vi "Cleanup.vi"(8 "error in (no error)":errorcluster, 11 "LabBOT in":refnum<class "LabBOT.lvclass">) -> (0 "error out":errorcluster)   [LabVIEW 2020, in "Rover.lvlib" / "LabBOT.lvclass"]
uses:
  LabBOT.lvclass
  LabBOT.lvclass/LabBOT.ctl
  Rover/Rover.lvclass
  nmea/nmea/VISA GPS/VISA GPS.lvclass
  bno055/BNO055/BNO055/BNO055.lvclass
  <vilib>/MakerHub/LINX/LMH-LINX.lvlib
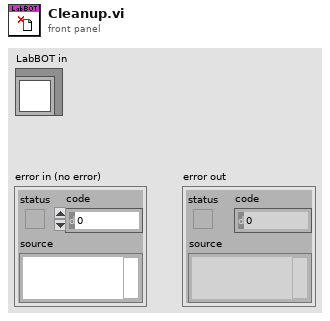
[diagram p1: front panel]
types:
  T1 = typedef "LMH-LINX.lvlib/LINX Ref.ctl" = cluster{"IO":T2, "Interface":T3, "LINX Device Config":T4}
  T2 = typedef "LMH-LINX.lvlib/Platform.ctl" = enum16{"Remote", "Local"}
  T3 = typedef "LMH-LINX.lvlib/Interface.ctl" = enum16{"Serial", "TCP"}
  T4 = typedef "LMH-LINX.lvlib/Device.lvlib/LINX Device Config.ctl" = cluster{"Interface":T3, "COM Port":refnum<visa-resource-name>, "TCP Configuration":T5, "Device Family":u8, "Device ID":u8, "Device Name":string, "TCP Ref":refnum<k5>, "Channels":T6}
  T5 = typedef "LMH-LINX.lvlib/Device.lvlib/TCP Config.ctl" = cluster{"IP Address":string, "Port":u16}
  T6 = typedef "LMH-LINX.lvlib/Channels.ctl" = cluster{"DI":u8[], "DO":u8[], "AI":u8[], "AO":u8[], "PWM":u8[], "QE":u8[], "UART":u8[], "I2C 2":u8[], "SPI":u8[], "CAN":u8[], "Servo":u8[], "AI Ref (V)":dbl, "AI Resolution (Bits)":u8, "AO Ref (V)":dbl, "AO Resolution (Bits)":u8}
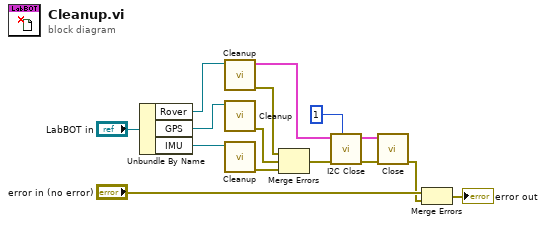
[diagram p0: block diagram]
diagram:
  n1 = Unbundle By Name("LabBOT in") -> ("Rover"=w13:refnum<class "Rover.lvclass">, "GPS"=w12:refnum<class "VISA GPS.lvclass">, "IMU"=w11:refnum<class "BNO055.lvclass">)
  n2 = call "Cleanup.vi"("Rover in"=w13) -> ("error out"=w8:errorcluster, "LINX Resource"=w6:T1)  [unwired: 9 in]
  n3 = call "Cleanup.vi"("VISA GPS in"=w12) -> ("error out"=w9:errorcluster)  [unwired: 10 in]
  n4 = call "Cleanup.vi"("BNO055 in"=w11) -> ("error out"=w10:errorcluster)  [unwired: 9 in, 1 out]
  n5 = Merge Errors(w8, w9, w10) -> (w7:errorcluster)
  n6 = call <vilib>:"I2C Close.vi"("I2C Channel (0)"=u8 1, "Error In"=w7, "LINX Resource"=w6) -> ("Error Out"=w4:errorcluster, "LINX Resource"=w3:T1)  [unwired: 7 in]
  n7 = call <vilib>:"Close.vi"("Error In"=w4, "LINX Resource"=w3) -> ("Error Out"=w1:errorcluster)  [unwired: 9 in]
  n8 = Merge Errors("error in (no error)", w1) -> (→"error out":errorcluster)
